vi "__keysight_setup.vi"(0 "Ouput 1":bool=TRUE, 1 "Frequency 1 (MHz)":dbl=10.0 min=0.0 max=14.5, 5 "Ouput 2":bool=TRUE, 7 "Ouput 1 Neg":bool=TRUE, 9 "Ouput 2 Neg":bool=TRUE, 11 "error in":errorcluster, 12 "Frequency 2 (MHz)":dbl=10.0 min=0.0 max=14.5) -> (4 "Command":string=":track:channel1 ON\n:frequency1 7.000MHz\n:output1 OFF\n:output2 OFF\n:output1:complement ON\n:output2:complement ON\n:output1:strobe:route NONE\n:output2:strobe:route NONE\n:output1:trigger:route SYNA\n:output2:trigger:route SYNB\n", 15 "error out":errorcluster)   [LabVIEW 2013]
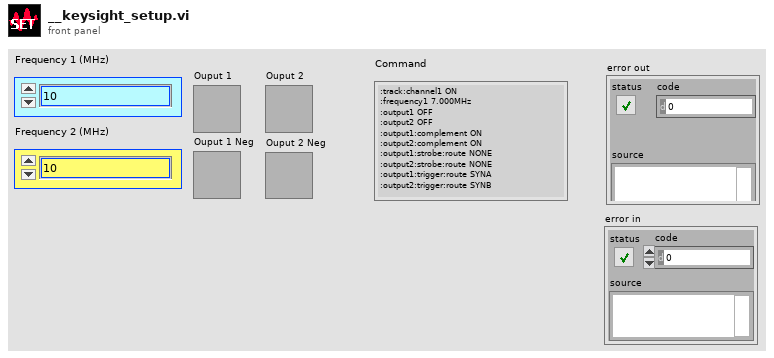
[diagram p1: front panel]
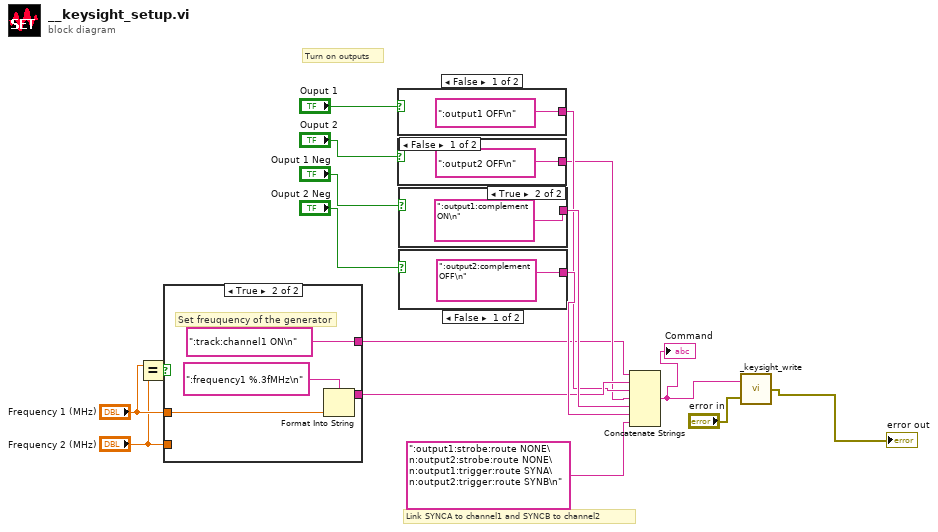
[diagram p0: block diagram]
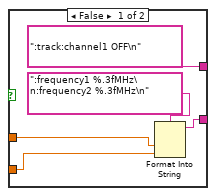
[diagram p2: hidden frame]
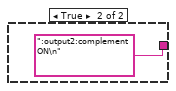
[diagram p3: hidden frame]
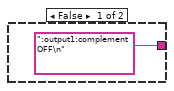
[diagram p4: hidden frame]
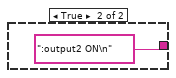
[diagram p5: hidden frame]
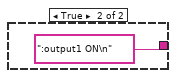
[diagram p6: hidden frame]
diagram:
  # "Link SYNCA to channel1 and SYNCB to channel2"
  # "Turn on outputs"
  n1 = Equal?(x="Frequency 1 (MHz)", y="Frequency 2 (MHz)") -> (x = y?=w7:bool)
  n2 = case shown="True" w7 {
    tunnel: "Frequency 1 (MHz)" -> [w21 w25]
    tunnel: [w19 w24] -> w11
    tunnel: "Frequency 2 (MHz)" -> [w20 _]
    tunnel: [":track:channel1 OFF\n" ":track:channel1 ON\n"] -> w2
    frame False {
      n3 = Format Into String(format string=":frequency1 %.3fMHz\n:frequency2 %.3fMHz\n", w21, w20) -> (resulting string=w19:string)  [unwired: 2 in, 1 out]
    }
    frame True {
      # "Set freuquency of the generator"
      n4 = Format Into String(format string=":frequency1 %.3fMHz\n", w25) -> (resulting string=w24:string)  [unwired: 2 in, 1 out]
    }
  }
  n5 = case shown="False" "Ouput 1" {
    tunnel: [":output1 OFF\n" ":output1 ON\n"] -> w10
    frame False {
    }
    frame True {
    }
  }
  n6 = case shown="False" "Ouput 2" {
    tunnel: [":output2 OFF\n" ":output2 ON\n"] -> w9
    frame False {
    }
    frame True {
    }
  }
  n7 = case shown="True" "Ouput 1 Neg" {
    tunnel: [":output1:complement OFF\n" ":output1:complement ON\n"] -> w13
    frame False {
    }
    frame True {
    }
  }
  n8 = case shown="False" "Ouput 2 Neg" {
    tunnel: [":output2:complement OFF\n" ":output2:complement ON\n"] -> w12
    frame False {
    }
    frame True {
    }
  }
  n9 = Concatenate Strings(w2, w11, w10, w9, w13, w12, ":output1:strobe:route NONE\n:output2:strobe:route NONE\n:output1:trigger:route SYNA\n:output2:trigger:route SYNB\n") -> (w1:string)
  "Command" <- w1
  n10 = call "_keysight_write.vi"("error in"="error in", "command"=w1) -> ("error out"=→"error out":errorcluster)
